vi "Configure Basic THD.vi"(6 "Fixed Frequency (10 Hz)":dbl=10.0, 7 "Tuning Source (0: tsMeasFreq)":i32(ring) items=["tsMeasFreq", "tsAnlgGenA", "tsAnlgGenB", "tsDigGenA", "tsDigGenB", "tsSweepSrc0", "tsSweepSrc1"], 8 "error in (no error)":errorcluster, 9 "Tuning Mode (0: tmFixed)":i32(ring) items=["tmFixed", "tmTuned"], 10 "Analyzer (0: A0)":i32(ring) items=["A0", "A1"], 11 "VISA resource name":refnum<visa-resource-name>) -> (0 "error out":errorcluster, 3 "VISA resource name out":refnum<visa-resource-name>)   [LabVIEW 2014, in "Stanford Research SR1.lvlib"]
doc: "Configure the basic attributes for the THD Analyzer."
uses:
  Stanford Research SR1.lvlib
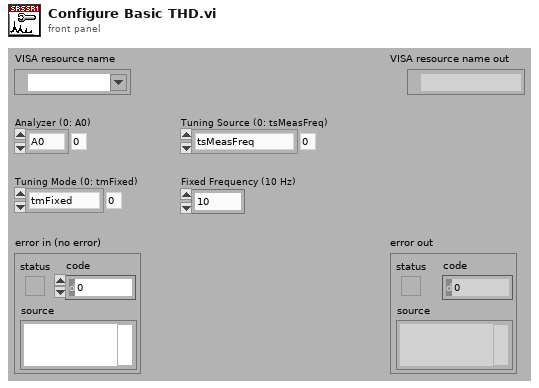
[diagram p1: front panel]
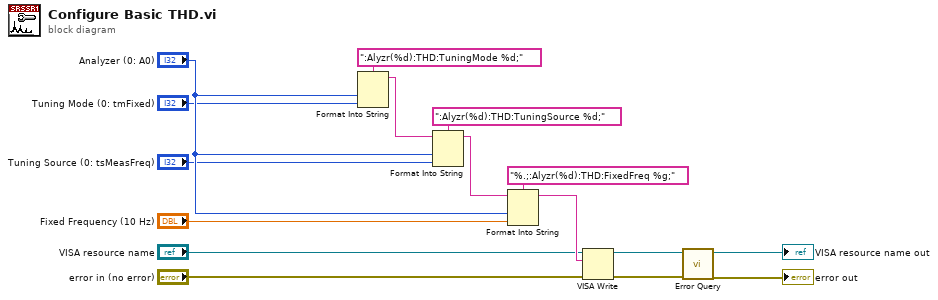
[diagram p0: block diagram]
diagram:
  n1 = Format Into String(format string=":Alyzr(%d):THD:TuningMode %d;", "Analyzer (0: A0)", "Tuning Mode (0: tmFixed)") -> (resulting string=w15:string)  [unwired: 2 in, 1 out]
  n2 = Format Into String(format string=":Alyzr(%d):THD:TuningSource %d;", initial string=w15, "Analyzer (0: A0)", "Tuning Source (0: tsMeasFreq)") -> (resulting string=w13:string)  [unwired: 1 in, 1 out]
  n3 = Format Into String(format string="%.;:Alyzr(%d):THD:FixedFreq %g;", initial string=w13, "Analyzer (0: A0)", "Fixed Frequency (10 Hz)") -> (resulting string=w11:string)  [unwired: 1 in, 1 out]
  n4 = VISA Write(VISA resource name="VISA resource name", write buffer=w11, error in (no error)="error in (no error)") -> (VISA resource name out=w8:refnum<visa-resource-name>, error out=w7:errorcluster)  [unwired: 1 out]
  n5 = call "Error Query.vi"("error in (no error)"=w7, "VISA resource name"=w8) -> ("error out"=→"error out":errorcluster, "VISA resource name out"=→"VISA resource name out":refnum<visa-resource-name>)  [unwired: 6 in, 2 out]
